vi "Rename.vi"(8 "error in (no error)":errorcluster, 9 "New FileName":string, 10 "File To Rename":string, 11 "FTP in":refnum<class "FTP.lvclass">) -> (0 "error out":errorcluster, 3 "FTP out":refnum<class "FTP.lvclass">)   [LabVIEW 2013, in "FTP.lvlib" / "FTP.lvclass"]
doc: "This vi will rename a file on the remote ftp server with the new name specified in the \"New FileName\" parameter."
uses:
  FTP.lvclass
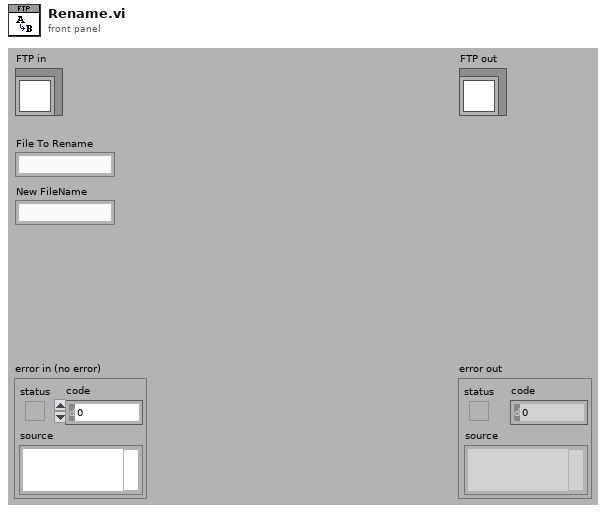
[diagram p1: front panel]
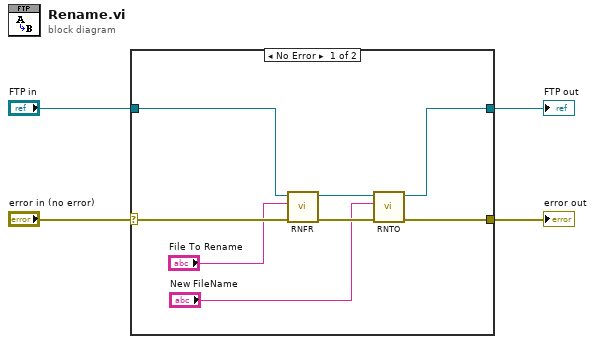
[diagram p0: block diagram]
diagram:
  n1 = case shown="No Error" "error in (no error)" {
    selector: "error in (no error)" -> [w9 w14]
    tunnel: [w7 w14] -> w3
    tunnel: [w10 w13] -> w1
    tunnel: "FTP in" -> [w12 w13]
    frame No Error {
      n2 = call "RNFR.vi"("error in (no error)"=w9, "File To Rename"="File To Rename", "FTP in"=w12) -> ("error out"=w8:errorcluster, "FTP out"=w11:refnum<class "FTP.lvclass">)  [unwired: 7 in]
      n3 = call "RNTO.vi"("error in (no error)"=w8, "New FileName"="New FileName", "FTP in"=w11) -> ("error out"=w7:errorcluster, "FTP out"=w10:refnum<class "FTP.lvclass">)  [unwired: 7 in]
    }
    frame Error {
    }
  }
  "error out" <- w3
  "FTP out" <- w1
